vi "Run.vi"(8 "error in (no error)":errorcluster, 11 "PmuBase in":refnum<class "PmuBase.lvclass">) -> (0 "error out":errorcluster, 1 "DataValid":bool, 2 "clSensorData":T1, 3 "PmuBase out":refnum<class "PmuBase.lvclass">)   [LabVIEW 2018, in "SensorPlugins.lvlib" / "PmuBase.lvclass"]
uses:
  PmuBase.lvclass
  SensorModule/PublicAPI/Arguments/Broadcasts/clSensorData.ctl
  SensorBaseClass/SensorBase.lvclass
  SensorShared/SensorShared.lvlib
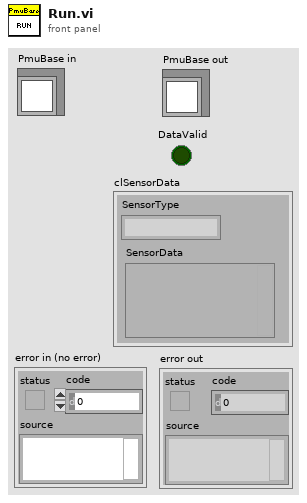
[diagram p1: front panel]
types:
  T1 = typedef "SensorShared.lvlib/clSensorData.ctl" = cluster{"SensorType":string, "SensorData":variant}
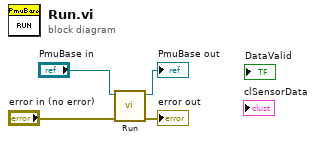
[diagram p0: block diagram]
diagram:
  n1 = call-parent "Run.vi"("error in (no error)"="error in (no error)", "SensorBase in"="PmuBase in") -> ("error out"=→"error out":errorcluster, "SensorBase out"=→"PmuBase out":refnum<class "PmuBase.lvclass">)  [unwired: 6 in, 2 out]
